vi "LoadTagConfiguration.vi"(2 "error in":errorcluster, 3 "AppName":string="LabWinders", 4 "XML Filename":string) -> (0 "error out":errorcluster, 1 "CVT Tag List":T1[](array[typedef]))   [LabVIEW 2018]
uses:
  <vilib>/NI/Current Value Table/Compatibility/_SubVIs/TypeDefs/cvt_Tag Configuration.ctl
  <vilib>/NI/Current Value Table/Compatibility/_SubVIs/TypeDefs/cvt_Data Types.ctl
  <vilib>/Utility/sysdir.llb/System Directory Type.ctl
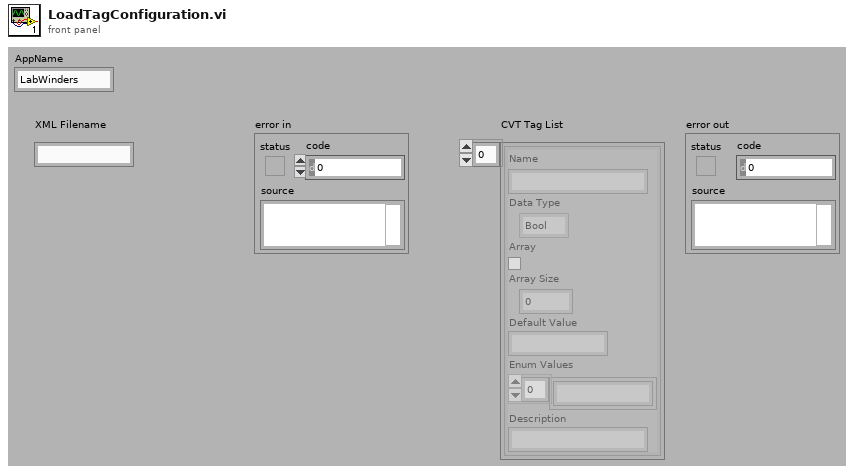
[diagram p1: front panel]
types:
  T1 = typedef "cvt_Tag Configuration.ctl" = cluster{"Name":string, "Data Type":T2, "Array":bool, "Size":u32, "Default":string, "Enum":string[], "Description":string}
  T2 = typedef "cvt_Data Types.ctl" = enum16{"Bool", "U8", "I32", "Double", "String", "Enum"}
  T3 = typedef "System Directory Type.ctl" = i32
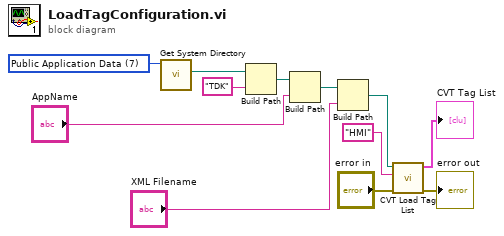
[diagram p0: block diagram]
diagram:
  w6 = T3 7 items=["User Home", "User Desktop", "User Documents", "User Application Data", "User Preferences", "User Temporary", "Public Documents", "Public Application Data", "Public Preferences", "System Core Libraries", "System Installed Libraries", "Application Files", "Boot Volume Root"] ("system directory type")
  n1 = call <vilib>:"Get System Directory.vi"("system directory type"=w6) -> ("system directory"=w7:path)  [unwired: 10 in]
  n2 = Build Path(base path=w7, name or relative path="TDK") -> (appended path=w9:path)
  n3 = Build Path(base path=w9, name or relative path="AppName") -> (appended path=w11:path)
  n4 = Build Path(base path=w11, name or relative path="XML Filename") -> (appended path=w5:path)
  n5 = call <vilib>:"CVT Load Tag List.vi"("error in"="error in", "Target Name"="HMI", "TCE Config File Path"=w5) -> ("error out"=→"error out":errorcluster, "CVT Tag List"=→"CVT Tag List":T1[])  [unwired: 7 in]
